vi "motortestMeng1.vi"() -> ()   [LabVIEW 2014]
panel:
  out "GetPosition":i32
  out "pfPosition":sgl
  out "Numeric":i32
  in  "Controller ID":i32=83829798
  in  "stop":bool
  in  "MG17Motor":refnum<k7>(container)
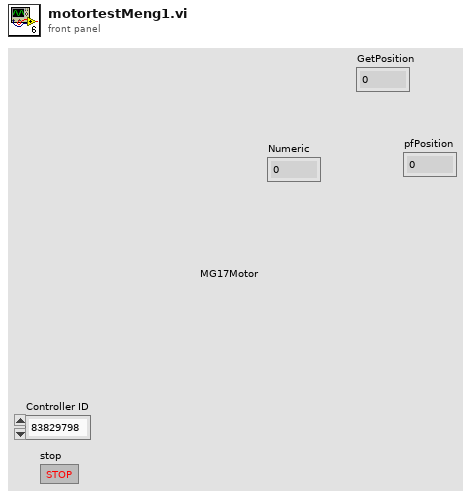
[diagram p1: front panel]
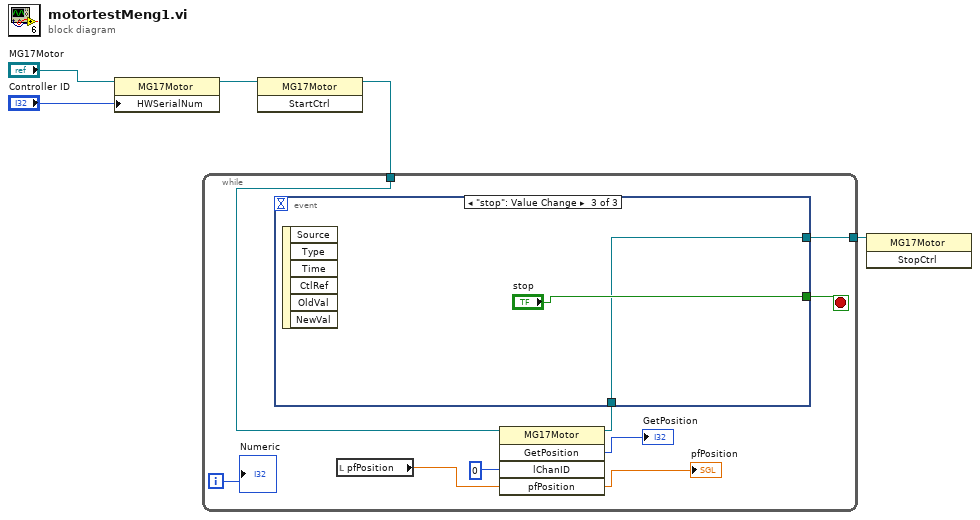
[diagram p0: block diagram]
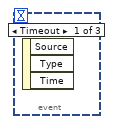
[diagram p2: hidden frame]
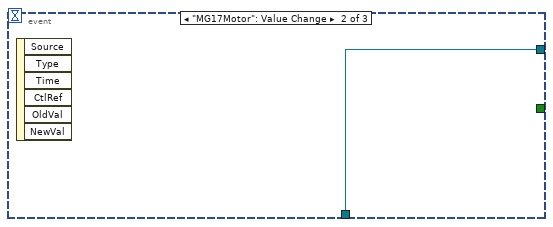
[diagram p3: hidden frame]
diagram:
  n1 = property class="MG17Motor"(reference="MG17Motor", "HWSerialNum"="Controller ID") -> (reference out=w3:refnum<k7>)  [unwired: 1 in, 1 out]
  n2 = invoke class="MG17Motor" method="StartCtrl"(reference=w3) -> (reference out=w2:refnum<k7>)  [unwired: 2 in, 2 out]
  n3 = while {
    tunnel: [w13] -> w5
    tunnel: w2 -> [w6]
    i -> [w14]
    stop <- w12 stop-if-true
    n4 = local read "pfPosition"() -> (w8:sgl)
    n5 = invoke class="MG17Motor" method="GetPosition"(reference=w6, "lChanID"=0, "pfPosition"=w8) -> (reference out=w7:refnum<k7>, "GetPosition"=→"GetPosition":i32, "pfPosition"=→"pfPosition":sgl)  [unwired: 2 in, 2 out]
    n6 = event shown="[2] \"stop\": Value Change" {
      selector: _ -> [_ _ _]
      dyn-events: _ -> [_ _ _]
      timeout: _ -> [_ _ _]
      tunnel: [_ w15 w16] -> w13
      tunnel: [_ _ "stop"] -> w12
      tunnel: w7 -> [_ w15 w16]
      event Timeout {
        n7 = event-data() -> ()  [unwired: 1 in, 3 out]
      }
      event "MG17Motor": Value Change {
        n8 = event-data() -> ()  [unwired: 1 in, 6 out]
      }
      event "stop": Value Change {
        n9 = event-data() -> ()  [unwired: 1 in, 6 out]
      }
    }
    "Numeric" <- w14
  }
  n10 = invoke class="MG17Motor" method="StopCtrl"(reference=w5) -> ()  [unwired: 2 in, 3 out]
